vi "Write Roundng Radius.vi"(8 "error in (no error)":errorcluster, 10 "Roundng Radius":dbl=15.0, 11 "RoundBouy in":refnum<class "RoundBouy.lvclass">) -> (0 "error out":errorcluster, 3 "RoundBouy out":refnum<class "RoundBouy.lvclass">)   [LabVIEW 2013, in "RoundBouy.lvclass"]
uses:
  RoundBouy.lvclass
  RoundBouy.lvclass/RoundBouy.ctl
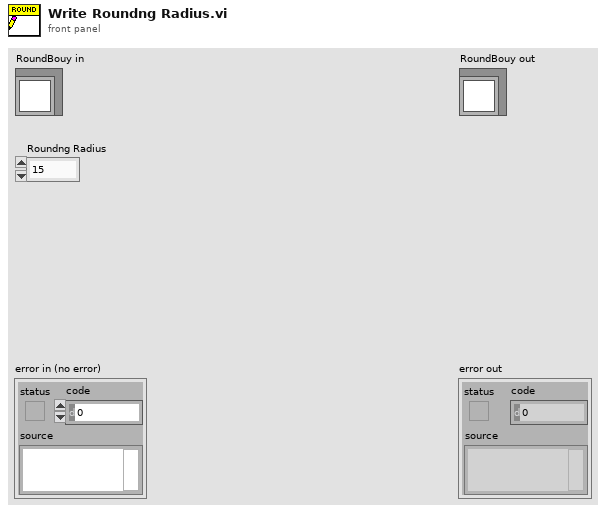
[diagram p1: front panel]
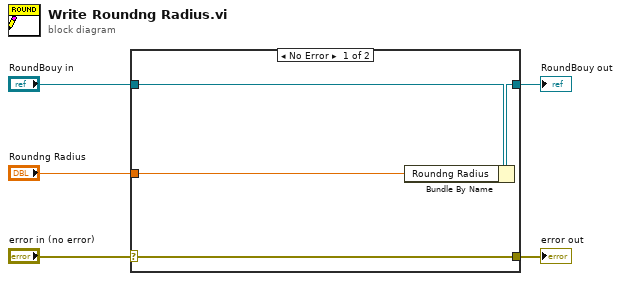
[diagram p0: block diagram]
diagram:
  n1 = case shown="No Error" "error in (no error)" {
    selector: "error in (no error)" -> [w9 w10]
    tunnel: [w9 w10] -> w4
    tunnel: [w7 w11] -> w2
    tunnel: "RoundBouy in" -> [w8 w11]
    tunnel: "Roundng Radius" -> [w6 _]
    frame No Error {
      n2 = Bundle By Name(cluster=w8, "Roundng Radius"=w6) -> (w7:refnum<class "RoundBouy.lvclass">)
    }
    frame Error {
    }
  }
  "error out" <- w4
  "RoundBouy out" <- w2
